vi "Listen Port.vi"(9 "Port in":u16=8080, 10 "Mode (Get Port)":enum16{"Init", "Get Port", "Set Port"}(ring)=enum."Get Port", 11 "Config File":path) -> (1 "Port out":u16)   [LabVIEW 2023]
doc: "This VIG acts as a helper to hold the Listening Port, including the ability to serialize/deserialize to an INI file."
uses:
  <vilib>/Utility/config.llb/Read Key (U32).vi
  <vilib>/Utility/config.llb/Write Key (U32).vi
  <vilib>/Utility/config.llb/NI_LVConfig.lvlib
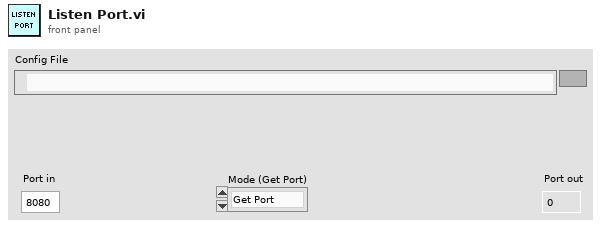
[diagram p1: front panel]
types:
  T1 = typedef "NI_LVConfig.lvlib/Config Data RefNum.ctl" = refnum<k1>
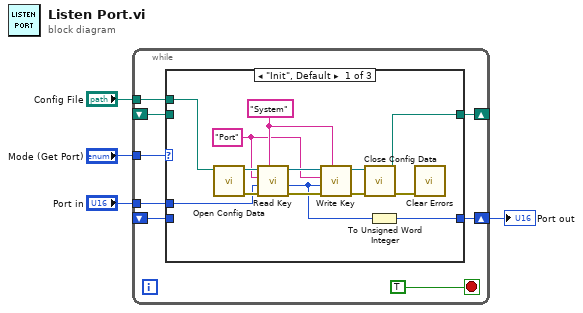
[diagram p0: block diagram]
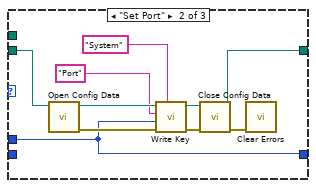
[diagram p2: hidden frame]
diagram:
  n1 = while {
    tunnel: "Mode (Get Port)" -> [w11]
    shift-right: [w8] -> w2
    shift-left: _ -> [w6]
    shift-right: [w10] -> _
    shift-left: _ -> [w7]
    tunnel: "Config File" -> [w9]
    tunnel: "Port in" -> [w5]
    stop <- TRUE stop-if-true
    n2 = case shown="\"Init\", Default" w11 {
      tunnel: [w17 w30 w38] -> w10
      tunnel: w9 -> [w18 _ _]
      tunnel: [w13 w29 w37] -> w8
      tunnel: w7 -> [_ w28 w38]
      tunnel: w6 -> [_ _ w37]
      tunnel: w5 -> [w14 w29 _]
      frame "Init", Default {
        w19 = "Port" ("section")
        w20 = "System" ("section")
        n3 = call <vilib>:"Open Config Data.vi"("configuration file path"=w18) -> ("error out"=w26:errorcluster, "refnum"=w24:T1)  [unwired: 8 in, 1 out]
        n4 = call-poly <vilib>:"Read Key.vi"("section"=w20, "error in (no error)"=w26, "default value"=w14, "key"=w19, "refnum"=w24) -> ("error out"=w25:errorcluster, "value"=w16:u32, "refnum out"=w22:T1)  [unwired: 3 in, 1 out]
        n5 = call-poly <vilib>:"Write Key.vi"("section"=w20, "error in (no error)"=w25, "value"=w16, "key"=w19, "refnum"=w22) -> ("error out"=w23:errorcluster, "refnum out"=w21:T1)  [unwired: 4 in, 1 out]
        n6 = call <vilib>:"Close Config Data.vi"("error in (no error)"=w23, "refnum"=w21) -> ("error out"=w15:errorcluster, "file path"=w17:path)  [unwired: 8 in]
        n7 = To Unsigned Word Integer(number=w16) -> (unsigned 16bit integer=w13:u16)
        n8 = call <vilib>:"Clear Errors.vi"("error in (no error)"=w15) -> ()  [unwired: 5 in, 2 out]
      }
      frame "Set Port" {
        n9 = call <vilib>:"Open Config Data.vi"("configuration file path"=w28) -> ("error out"=w36:errorcluster, "refnum"=w34:T1)  [unwired: 8 in, 1 out]
        n10 = call-poly <vilib>:"Write Key.vi"("section"="System", "error in (no error)"=w36, "value"=w29, "key"="Port" ("section"), "refnum"=w34) -> ("error out"=w35:errorcluster, "refnum out"=w33:T1)  [unwired: 4 in, 1 out]
        n11 = call <vilib>:"Close Config Data.vi"("error in (no error)"=w35, "refnum"=w33) -> ("error out"=w27:errorcluster, "file path"=w30:path)  [unwired: 8 in]
        n12 = call <vilib>:"Clear Errors.vi"("error in (no error)"=w27) -> ()  [unwired: 5 in, 2 out]
      }
      frame "Get Port" {
      }
    }
  }
  "Port out" <- w2
